vi "Configure Capacitor C1.vi"(8 "error in (no error)":errorcluster, 10 "position, %":u8, 11 "MKS MW in":refnum<class "PL MKS MW.lvclass">) -> (0 "error out":errorcluster, 3 "MKS MW out":refnum<class "PL MKS MW.lvclass">)   [LabVIEW 2015, in "PL MKS MW.lvclass"]
doc: "Configures capacitor C1 <b>position</b>."
uses:
  PL MKS MW.lvclass
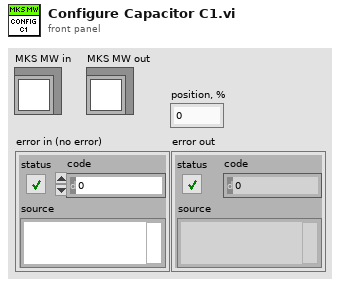
[diagram p1: front panel]
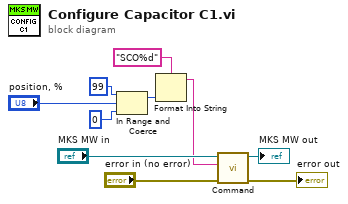
[diagram p0: block diagram]
diagram:
  n1 = In Range and Coerce(upper limit=u8 99, x="position, %", lower limit=u8 0) -> (coerced(x)=w2:u8)  [unwired: 1 out]
  n2 = Format Into String(format string="SCO%d", w2) -> (resulting string=w1:string)  [unwired: 2 in, 1 out]
  n3 = call "Command.vi"("error in (no error)"="error in (no error)", "command"=w1, "MKS MW in"="MKS MW in") -> ("error out"=→"error out":errorcluster, "MKS MW out"=→"MKS MW out":refnum<class "PL MKS MW.lvclass">)  [unwired: 6 in, 1 out]
